vi "CMD_ACKFAULT.vi"(6 "Gantry in":refnum<class "Gantry.lvclass">, 8 "error in (no error)":errorcluster, 10 "Arguments":string[](array[string]), 11 "gScript Interpreter in":refnum<class "gScript Interpreter.lvclass">) -> (0 "error out":errorcluster, 3 "gScript Interpreter out":refnum<class "gScript Interpreter.lvclass">, 4 "Gantry out":refnum<class "Gantry.lvclass">)   [LabVIEW 2017, in "gScript Interpreter.lvclass"]
uses:
  gScript Interpreter.lvclass
  Shared Components/Gantry Class/Gantry.lvclass
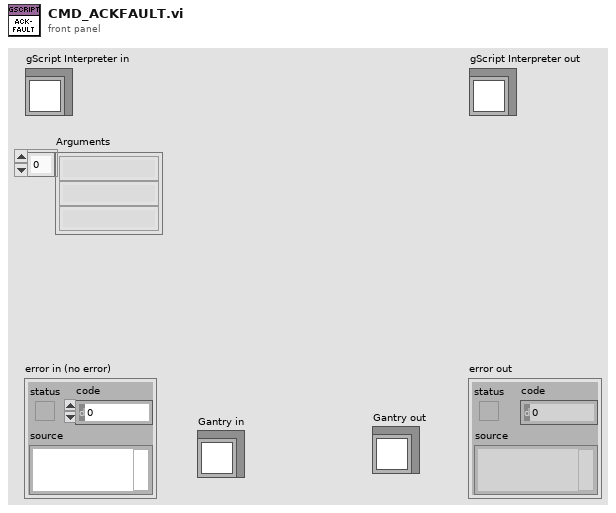
[diagram p1: front panel]
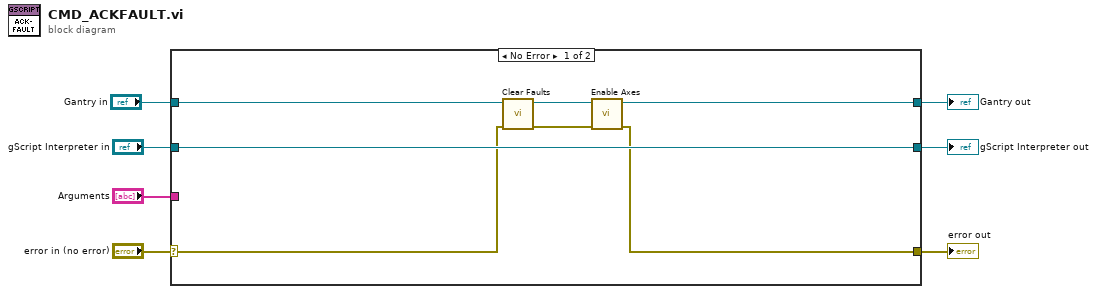
[diagram p0: block diagram]
diagram:
  n1 = case shown="No Error" "error in (no error)" {
    selector: "error in (no error)" -> [w12 w17]
    tunnel: [w8 w17] -> w6
    tunnel: [w14 w16] -> w4
    tunnel: "gScript Interpreter in" -> [w14 w16]
    tunnel: "Arguments" -> [_ _]
    tunnel: "Gantry in" -> [w13 w15]
    tunnel: [w10 w15] -> w1
    frame No Error {
      n2 = call-dynamic "Clear Faults.vi"("error in"=w12, "Gantry in"=w13) -> ("error out"=w9:errorcluster, "Gantry out"=w11:refnum<class "Gantry.lvclass">)  [unwired: 8 in]
      n3 = call-dynamic "Enable Axes.vi"("error in"=w9, "Gantry in"=w11) -> ("error out"=w8:errorcluster, "Gantry out"=w10:refnum<class "Gantry.lvclass">)  [unwired: 8 in]
    }
    frame Error {
    }
  }
  "error out" <- w6
  "gScript Interpreter out" <- w4
  "Gantry out" <- w1
